vi "E13_Semaforo_case_array_Arduino.vi"() -> ()   [LabVIEW 2020]
uses:
  <vilib>/MakerHub/LINX/Public/Peripherals/Digital/Digital Write N Chans.vi
  <vilib>/MakerHub/LINX/Private/Local IO/LinxDigitalWrite.vi
  <vilib>/MakerHub/LINX/Public/Utilities/Check Channel.vi
  <vilib>/MakerHub/LINX/Public/Utilities/Open Serial.vi
  <vilib>/MakerHub/LINX/Private/Utilties/Generate Error.vi
  <vilib>/MakerHub/LINX/LMH-LINX.lvlib
panel:
  in  "Serial Port":refnum<visa-resource-name>="N/A"
  out "V3":bool
  out "A3":bool
  out "R3":bool
  out "Seq 2":i32
  out "V4":bool
  out "A4":bool
  out "R4":bool
  in  "stop 2":bool
  in  "stop":bool
  out "R2":bool
  out "A2":bool
  out "V2":bool
  out "Seq":i32
  out "R1":bool
  out "A1":bool
  out "V1":bool
  # "Array with Arduino"
  # "Case"
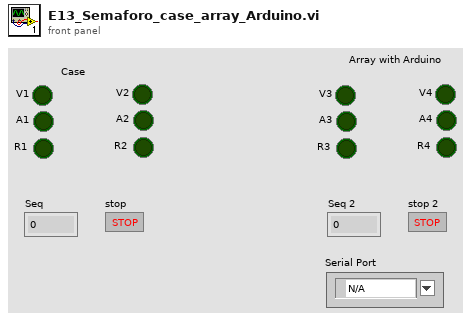
[diagram p1: front panel]
types:
  T1 = typedef "LMH-LINX.lvlib/LINX Ref.ctl" = cluster{"IO":T2, "Interface":T3, "LINX Device Config":T4}
  T2 = typedef "LMH-LINX.lvlib/Platform.ctl" = enum16{"Remote", "Local"}
  T3 = typedef "LMH-LINX.lvlib/Interface.ctl" = enum16{"Serial", "TCP"}
  T4 = typedef "LMH-LINX.lvlib/Device.lvlib/LINX Device Config.ctl" = cluster{"Interface":T3, "COM Port":refnum<visa-resource-name>, "TCP Configuration":T5, "Device Family":u8, "Device ID":u8, "Device Name":string, "TCP Ref":refnum<k5>, "Channels":T6}
  T5 = typedef "LMH-LINX.lvlib/Device.lvlib/TCP Config.ctl" = cluster{"IP Address":string, "Port":u16}
  T6 = typedef "LMH-LINX.lvlib/Channels.ctl" = cluster{"DI":u8[], "DO":u8[], "AI":u8[], "AO":u8[], "PWM":u8[], "QE":u8[], "UART":u8[], "I2C 2":u8[], "SPI":u8[], "CAN":u8[], "Servo":u8[], "AI Ref (V)":dbl, "AI Resolution (Bits)":u8, "AO Ref (V)":dbl, "AO Resolution (Bits)":u8}
  T7 = cluster{"[0]":bool, "[1]":bool, "[2]":bool, "[3]":bool, "[4]":bool, "[5]":bool, "[6]":bool, "[7]":bool, "[8]":bool}
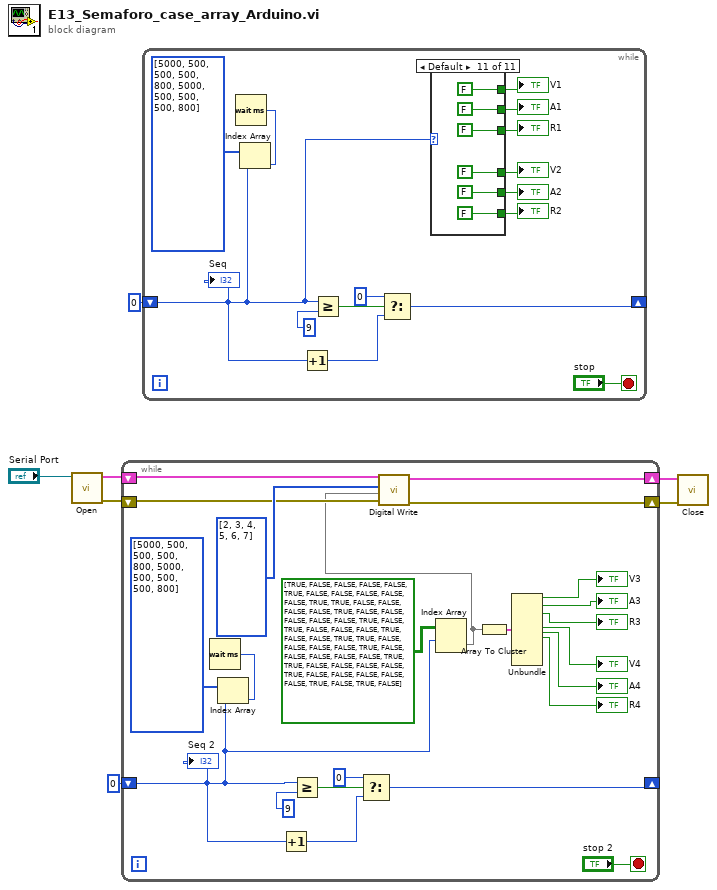
[diagram p0: block diagram]
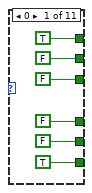
[diagram p2: hidden frame]
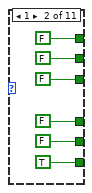
[diagram p3: hidden frame]
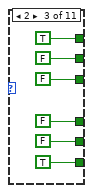
[diagram p4: hidden frame]
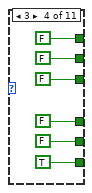
[diagram p5: hidden frame]
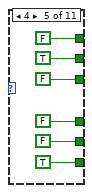
[diagram p6: hidden frame]
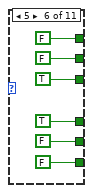
[diagram p7: hidden frame]
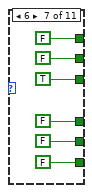
[diagram p8: hidden frame]
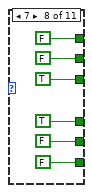
[diagram p9: hidden frame]
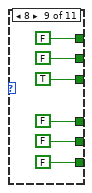
[diagram p10: hidden frame]
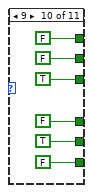
[diagram p11: hidden frame]
diagram:
  n1 = call-poly <vilib>:"Open.vi"("Serial Port"="Serial Port") -> ("Error Out"=w4:errorcluster, "LINX Resource"=w5:T1)  [unwired: 8 in, 1 out]
  n2 = while {
    shift-right: [w29] -> _
    shift-left: 0 -> [w14]
    shift-right: [w10] -> w3
    shift-left: w5 -> [w12]
    shift-right: [w9] -> w2
    shift-left: w4 -> [w11]
    stop <- "stop 2" stop-if-true
    n3 = Index Array(array=u32[] [5000, 500, 500, 500, 800, 5000, 500, 500, 500, 800], index=w14) -> (element=w24:u32)
    n4 = Wait (ms)(milliseconds to wait=w24) -> ()  [unwired: 1 out]
    n5 = Increment(x=w14) -> (x+1=w28:i32)
    n6 = Greater Or Equal?(x=w14, y=9) -> (x >= y?=w30:bool)
    n7 = Select(t=0, s=w30, f=w28) -> (s? t:f=w29:i32)
    n8 = Index Array(array=bool[][] [[TRUE, FALSE, FALSE, FALSE, FALSE, TRUE], [FALSE, FALSE, FALSE, FALSE, FALSE, TRUE], [TRUE, FALSE, FALSE, FALSE, FALSE, TRUE], [FALSE, FALSE, FALSE, FALSE, FALSE, TRUE], [FALSE, TRUE, FALSE, FALSE, FALSE, TRUE], [FALSE, FALSE, TRUE, TRUE, FALSE, FALSE], [FALSE, FALSE, TRUE, FALSE, FALSE, FALSE], [FALSE, FALSE, TRUE, TRUE, FALSE, FALSE], [FALSE, FALSE, TRUE, FALSE, FALSE, FALSE], [FALSE, FALSE, TRUE, FALSE, TRUE, FALSE]], index (row)=w14) -> (element=w8:bool[])  [unwired: 1 in]
    n9 = call-poly <vilib>:"Digital Write.vi"("Error In"=w11, "Values"=w8, "DO Channels"=u8[] [2, 3, 4, 5, 6, 7], "LINX Resource"=w12) -> ("Error Out"=w9:errorcluster, "LINX Resource"=w10:T1)  [unwired: 6 in]
    n10 = Array To Cluster(array=w8) -> (cluster=w22:T7)
    n11 = Unbundle(w22) -> ("[0]"=→"V3":bool, "[1]"=→"A3":bool, "[2]"=→"R3":bool, "[3]"=→"V4":bool, "[4]"=→"A4":bool, "[5]"=→"R4":bool)  [unwired: 3 out]
    "Seq 2" <- w14
  }
  n12 = while {
    shift-right: [w44] -> _
    shift-left: 0 -> [w31]
    stop <- "stop" stop-if-true
    n13 = Index Array(array=u32[] [5000, 500, 500, 500, 800, 5000, 500, 500, 500, 800], index=w31) -> (element=w33:u32)
    n14 = Wait (ms)(milliseconds to wait=w33) -> ()  [unwired: 1 out]
    n15 = Increment(x=w31) -> (x+1=w43:i32)
    n16 = Greater Or Equal?(x=w31, y=9) -> (x >= y?=w45:bool)
    n17 = Select(t=0, s=w45, f=w43) -> (s? t:f=w44:i32)
    n18 = case shown="Default" w31 {
      tunnel: [TRUE FALSE TRUE FALSE FALSE FALSE FALSE FALSE FALSE FALSE FALSE] -> w40
      tunnel: [FALSE FALSE FALSE FALSE TRUE FALSE FALSE FALSE FALSE FALSE FALSE] -> w39
      tunnel: [FALSE FALSE FALSE FALSE FALSE TRUE TRUE TRUE TRUE TRUE FALSE] -> w38
      tunnel: [FALSE FALSE FALSE FALSE FALSE TRUE FALSE TRUE FALSE FALSE FALSE] -> w37
      tunnel: [FALSE FALSE FALSE FALSE FALSE FALSE FALSE FALSE FALSE TRUE FALSE] -> w36
      tunnel: [TRUE TRUE TRUE TRUE TRUE FALSE FALSE FALSE FALSE FALSE FALSE] -> w35
      frame 0 {
      }
      frame 1 {
      }
      frame 2 {
      }
      frame 3 {
      }
      frame 4 {
      }
      frame 5 {
      }
      frame 6 {
      }
      frame 7 {
      }
      frame 8 {
      }
      frame 9 {
      }
      frame Default {
      }
    }
    "V1" <- w40
    "A1" <- w39
    "R1" <- w38
    "V2" <- w37
    "A2" <- w36
    "R2" <- w35
    "Seq" <- w31
  }
  n19 = call <vilib>:"Close.vi"("Error In"=w2, "LINX Resource"=w3) -> ()  [unwired: 9 in, 1 out]
